vi "Calculate Delay Time series.vi"(8 "error in (no error)":errorcluster, 11 "Readout Charact in":refnum<class "Readout Charact.lvclass">) -> (0 "error out":errorcluster, 3 "Readout Charact out":refnum<class "Readout Charact.lvclass">)   [LabVIEW 2018, in "Readout Charact.lvclass"]
uses:
  Readout Charact.lvclass
  CCDCamera/CCDCamera.lvclass
  LV2018/Interface/Interface.lvclass
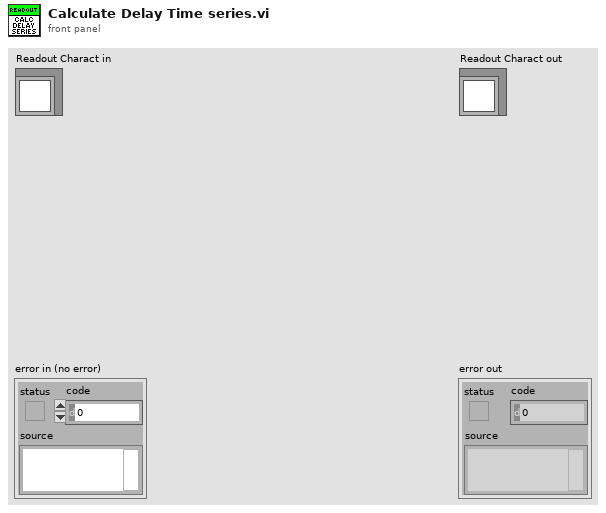
[diagram p1: front panel]
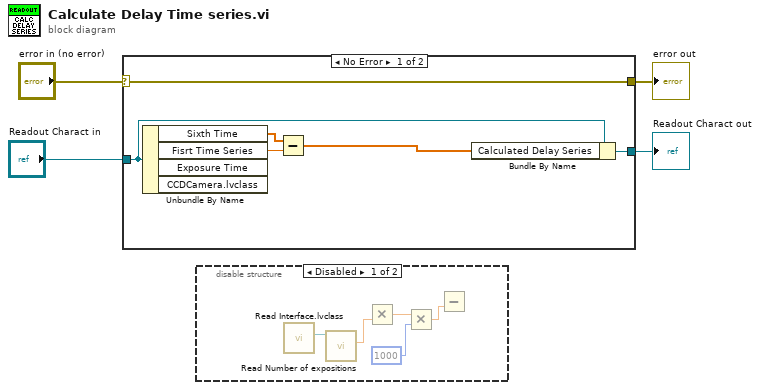
[diagram p0: block diagram]
diagram:
  n1 = case shown="No Error" "error in (no error)" {
    selector: "error in (no error)" -> [w10 w12]
    tunnel: [w10 w12] -> w3
    tunnel: [w6 w11] -> w1
    tunnel: "Readout Charact in" -> [w7 w11]
    frame No Error {
      n2 = Unbundle By Name(w7) -> ("Sixth Time"=w9:dbl[], "Fisrt Time Series"=w8:dbl)  [unwired: 2 out]
      n3 = Subtract(x=w9, y=w8) -> (x-y=w5:dbl[])
      n4 = Bundle By Name(cluster=w7, "Calculated Delay Series"=w5) -> (w6:refnum<class "Readout Charact.lvclass">)
    }
    frame Error {
    }
  }
  "error out" <- w3
  "Readout Charact out" <- w1
  n5 = disable-structure shown="Disabled" {
    frame Disabled {
      n6 = call-dynamic "Read Interface.lvclass.vi"() -> ("Interface.lvclass"=w14:refnum<class "Interface.lvclass">)  [unwired: 9 in, 2 out]
      n7 = call-dynamic "Read Number of expositions.vi"("Interface in"=w14) -> ("Number of expositions"=w16:dbl)  [unwired: 8 in, 2 out]
      n8 = Multiply(y=w16) -> (x=w15:dbl, x*y=w17:dbl)
      n9 = Multiply(x=w17, y=1000) -> (x*y=w13:dbl)
      n10 = Subtract(y=w13) -> ()  [unwired: 1 in, 1 out]
    }
    frame Enabled {
    }
  }
